vi "Out_S2F30.vi"(8 "error in (no error)":errorcluster, 10 "S2F30":T1, 11 "S2 Message Class in":refnum<class "S2 Message Class.lvclass">) -> (0 "error out":errorcluster, 3 "S2 Message Class out":refnum<class "S2 Message Class.lvclass">)   [LabVIEW 2020, in "SECS Communication.lvlib" / "S2 Message Class.lvclass"]
uses:
  S2 Message Class.lvclass
  D:/Dropbox/SECS/SECS_GEM v1.0.6/Com/SECS Communication/SECS-II Class/SECS-II Class.lvclass
  S2F30.ctl
  SECS-II Class/Data Message_List.vi
  SECS-II Class/Data Message_U4.vi
  SECS-II Class/Data Message_ASCII.vi
  SECS-II Class/SECS-II Class.lvclass
  D:/Dropbox/SECS/SECS_GEM v1.0.6/Com/SECS Communication/S2 Message Class/S2 Message Class.lvclass
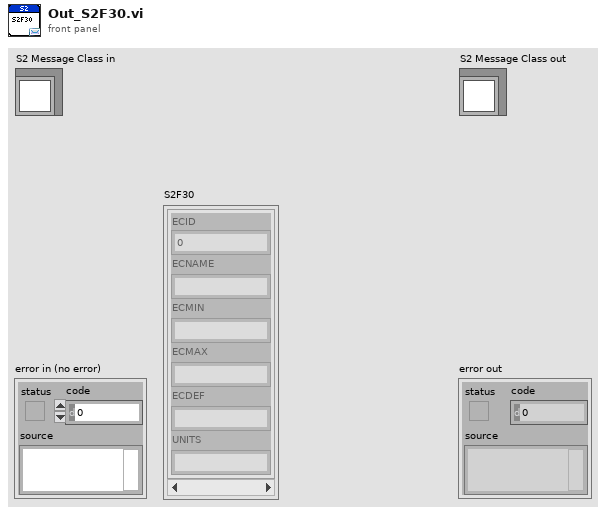
[diagram p1: front panel]
types:
  T1 = typedef "SECS Communication.lvlib/S2 Message Class.lvclass/S2F30.ctl" = cluster{"ECID":u32, "ECNAME":string, "ECMIN":string, "ECMAX":string, "ECDEF":string, "UNITS":string}[]
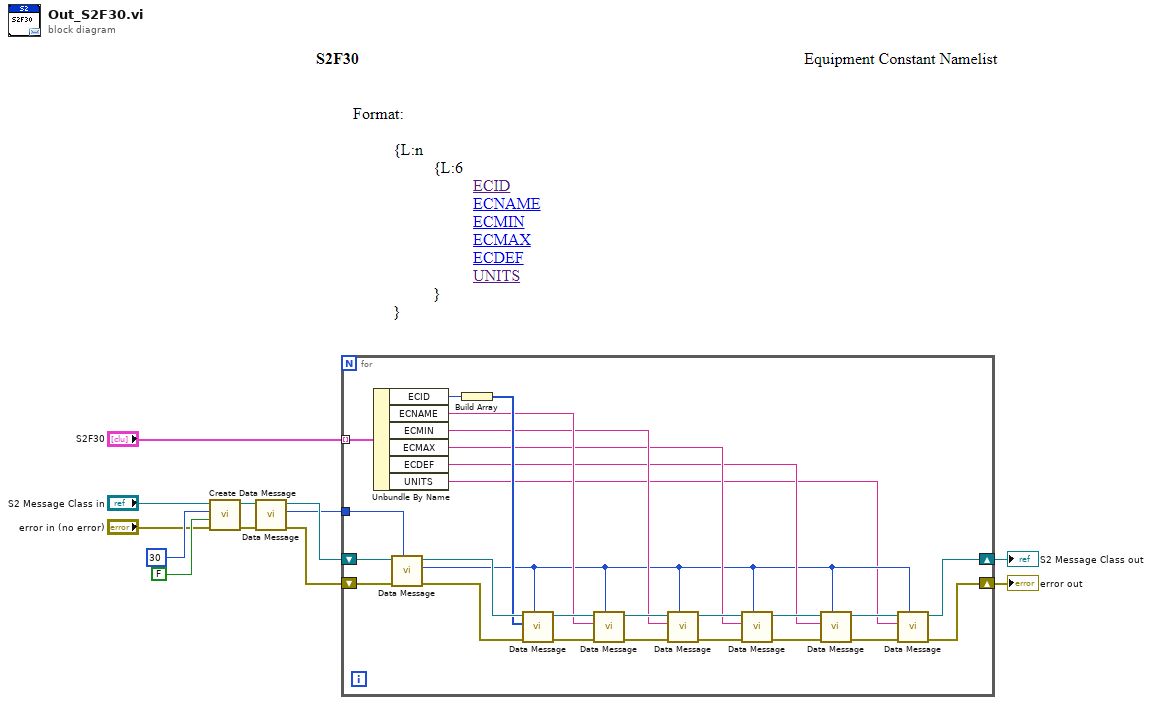
[diagram p0: block diagram]
diagram:
  n1 = call "Create Data Message.vi"("error in (no error)"="error in (no error)", "W-Bit"=FALSE, "Function"=u8 30, "SECS-II Class in"="S2 Message Class in") -> ("error out"=w7:errorcluster, "SECS-II Class out"=w6:refnum<class "S2 Message Class.lvclass">)  [unwired: 6 in]
  n2 = call-poly "Data Message.vi"("error in"=w7, "SECS-II Class in"=w6) -> ("error out"=w5:errorcluster, "Index"=w3:i32, "SECS-II Class out"=w4:refnum<class "S2 Message Class.lvclass">)  [unwired: 7 in]
  n3 = for {
    shift-right: [w14] -> w2
    shift-left: w4 -> [w38]
    shift-right: [w13] -> w1
    shift-left: w5 -> [w37]
    tunnel: "S2F30" -> [w33] mode=indexing
    tunnel: w3 -> [w34]
    n4 = Unbundle By Name(w33) -> ("ECID"=w32:u32, "ECNAME"=w28:string, "ECMIN"=w25:string, "ECMAX"=w22:string, "ECDEF"=w19:string, "UNITS"=w15:string)
    n5 = call-poly "Data Message.vi"("Parent Index"=w34, "error in"=w37, "SECS-II Class in"=w38) -> ("error out"=w36:errorcluster, "Index"=w16:i32, "SECS-II Class out"=w35:refnum<class "S2 Message Class.lvclass">)  [unwired: 6 in]
    n6 = Build Array(w32) -> (w31:u32[])
    n7 = call-poly "Data Message.vi"("Parent Index"=w16, "error in"=w36, "Data"=w31, "SECS-II Class in"=w35) -> ("error out"=w29:errorcluster, "SECS-II Class out"=w30:refnum<class "S2 Message Class.lvclass">)  [unwired: 6 in]
    n8 = call-poly "Data Message.vi"("Parent Index"=w16, "error in"=w29, "Data"=w28, "SECS-II Class in"=w30) -> ("error out"=w26:errorcluster, "SECS-II Class out"=w27:refnum<class "S2 Message Class.lvclass">)  [unwired: 6 in]
    n9 = call-poly "Data Message.vi"("Parent Index"=w16, "error in"=w26, "Data"=w25, "SECS-II Class in"=w27) -> ("error out"=w23:errorcluster, "SECS-II Class out"=w24:refnum<class "S2 Message Class.lvclass">)  [unwired: 6 in]
    n10 = call-poly "Data Message.vi"("Parent Index"=w16, "error in"=w23, "Data"=w22, "SECS-II Class in"=w24) -> ("error out"=w20:errorcluster, "SECS-II Class out"=w21:refnum<class "S2 Message Class.lvclass">)  [unwired: 6 in]
    n11 = call-poly "Data Message.vi"("Parent Index"=w16, "error in"=w20, "Data"=w19, "SECS-II Class in"=w21) -> ("error out"=w17:errorcluster, "SECS-II Class out"=w18:refnum<class "S2 Message Class.lvclass">)  [unwired: 6 in]
    n12 = call-poly "Data Message.vi"("Parent Index"=w16, "error in"=w17, "Data"=w15, "SECS-II Class in"=w18) -> ("error out"=w13:errorcluster, "SECS-II Class out"=w14:refnum<class "S2 Message Class.lvclass">)  [unwired: 6 in]
  }
  "error out" <- w1
  "S2 Message Class out" <- w2
